vi "ma_SML Peak-hold Averaging (complex input, scalar).vi"(0 "x":cdb format="%.2f", 1 "reset?":bool) -> (2 "y":cdb format="%.2f", 3 "averages sofar":dbl, 4 "data ready?":bool)   [LabVIEW 2020, in "NI_MAPro.lvlib"]
uses:
  NI_MAPro.lvlib
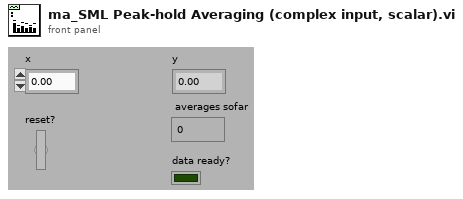
[diagram p1: front panel]
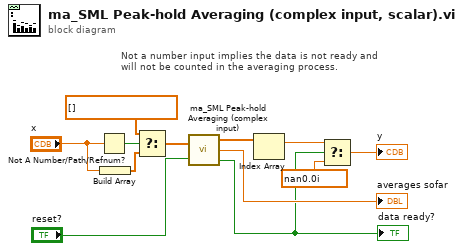
[diagram p0: block diagram]
diagram:
  # "Not a number input implies the data is not ready and \nwill not be counted in the averaging process."
  n1 = Not A Number/Path/Refnum?(number/path/refnum="x") -> (NaN/Path/Refnum?=w12:bool)
  n2 = Build Array("x") -> (w8:cdb[])
  n3 = Select(t=cdb[] [] ("x"), s=w12, f=w8) -> (s? t:f=w7:cdb[])
  n4 = call "ma_SML Peak-hold Averaging (complex input).vi"("x"=w7, "reset?"="reset?") -> ("y"=w6:cdb[], "averages sofar"=→"averages sofar":dbl, "data ready?"=w4:bool)
  "data ready?" <- w4
  n5 = Index Array(array=w6) -> (element=w3:cdb)  [unwired: 1 in]
  n6 = Select(t=w3, s=w4, f=cdb nan+0.0i) -> (s? t:f=→"y":cdb)
